vi "Robot Main.vi"() -> ()   [LabVIEW 2019]
doc: "This VI implements the framework and scheduler for your robotics program. It should not be necessary to modify the framework. You are expected to add your code to the VIs called from Robot Main - the ones located in the Team Code folder within the project."
uses:
  <vilib>/Rock Robotics/SystemInterfaces/i2clib/i2c_bus.ctl
panel:
  in  "Color":string(combo)="Red"
  in  "Set Color":bool
  out "Matched Color Name":string
  out "Match Confidence":dbl
  out "Measured Color":cluster{"R":dbl, "G":dbl, "B":dbl}
  in  "Blue Cal":cluster{"R":dbl, "G":dbl, "B":dbl}={"R"=0.143, "G"=0.427, "B"=0.429} caption="Blue Calibration"
  in  "Green Cal":cluster{"R":dbl, "G":dbl, "B":dbl}={"R"=0.197, "G"=0.561, "B"=0.24} caption="Green Calibration"
  in  "Red Cal":cluster{"R":dbl, "G":dbl, "B":dbl}={"R"=0.561, "G"=0.323, "B"=0.114} caption="Red Calibration"
  in  "Yellow Cal":cluster{"R":dbl, "G":dbl, "B":dbl}={"R"=0.361, "G"=0.524, "B"=0.113} caption="Yellow Calibration"
  out "error out":errorcluster
  out "Proximity":u16(graph)
  out "Color":u32(colorbox)
  in  "I2C Bus":T1
  in  "Finish":bool
  # "To save calibration:\n\nEdit --> Make Current Values Default"
  # "------>"
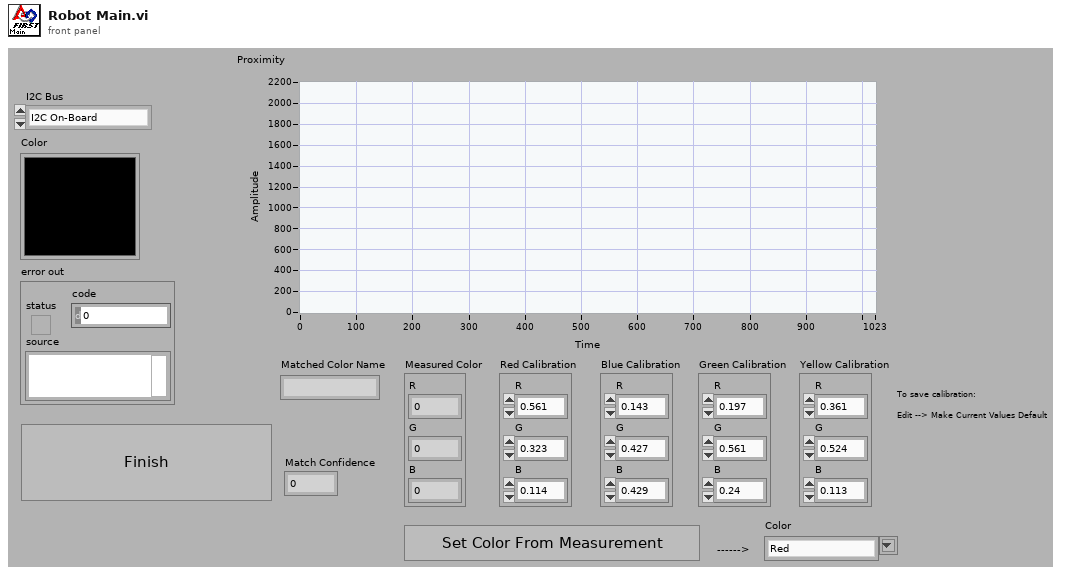
[diagram p1: front panel]
types:
  T1 = typedef "i2c_bus.ctl" = enum16{"I2C On-Board", "I2C MXP", "Invalid"}
  T2 = typedef "Color Sensor V3 DevRef.ctl" = cluster{"I2CDevRef":T3}
  T3 = typedef "WPI_I2CDevRef.ctl" = cluster{"DevStatus":errorcluster, "Device Address":u8, "Handle":i32, "I2C Bus":T1}
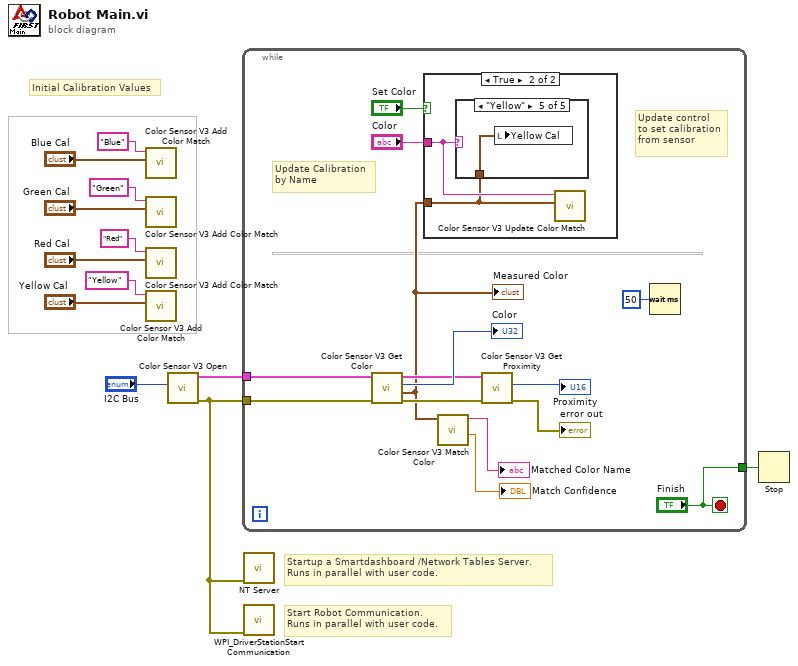
[diagram p0: block diagram]
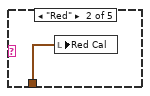
[diagram p4: hidden frame]
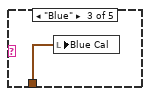
[diagram p5: hidden frame]
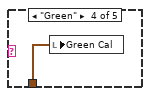
[diagram p6: hidden frame]
diagram:
  # "Initial Calibration Values"
  # "Startup a Smartdashboard /Network Tables Server.\nRuns in parallel with user code."
  # "Start Robot Communication.\nRuns in parallel with user code."
  n1 = call "Color Sensor V3 Add Color Match.vi"("Color"="Blue Cal", "Name"="Blue") -> ()  [unwired: 10 in]
  n2 = call "Color Sensor V3 Add Color Match.vi"("Color"="Green Cal", "Name"="Green") -> ()  [unwired: 10 in]
  n3 = call "Color Sensor V3 Add Color Match.vi"("Color"="Red Cal", "Name"="Red") -> ()  [unwired: 10 in]
  n4 = call "Color Sensor V3 Add Color Match.vi"("Color"="Yellow Cal", "Name"="Yellow") -> ()  [unwired: 10 in]
  n5 = call "Color Sensor V3 Open.vi"("I2C Bus"="I2C Bus") -> ("error out"=w10:errorcluster, "ColorSensorDevRef"=w11:T2)  [unwired: 9 in]
  n6 = while "Scheduling loop" {
    tunnel: w11 -> [w14]
    tunnel: w10 -> [w19]
    tunnel: ["Finish"] -> w9
    stop <- "Finish" stop-if-true
    # "Update control\nto set calibration\nfrom sensor"
    # "Update Calibration\nby Name"
    n7 = call "Color Sensor V3 Get Color.vi"("error in (no error)"=w19, "ColorSensorDevRef"=w14) -> ("error out"=w24:errorcluster, "Normalized Color"=w13:cluster{"R":dbl, "G":dbl, "B":dbl}, "Color"=→"Color":u32, "ColorSensorDevRef out"=w23:T2)  [unwired: 6 in]
    "Measured Color" <- w13
    n8 = case shown="True" "Set Color" {
      tunnel: "Color" -> [_ w28]
      tunnel: w13 -> [_ w27]
      frame False {
      }
      frame True {
        n9 = case shown="\"Yellow\"" w28 {
          tunnel: w27 -> [_ w29 w30 w31 w32]
          frame Default {
          }
          frame "Red" {
            n10 = local write "Red Cal"(w29) -> ()
          }
          frame "Blue" {
            n11 = local write "Blue Cal"(w30) -> ()
          }
          frame "Green" {
            n12 = local write "Green Cal"(w31) -> ()
          }
          frame "Yellow" {
            n13 = local write "Yellow Cal"(w32) -> ()
          }
        }
        n14 = call "Color Sensor V3 Update Color Match.vi"("Color"=w27, "Name"=w28) -> ()  [unwired: 10 in]
      }
    }
    n15 = call "Color Sensor V3 Match Color.vi"("Measured Color"=w13) -> ("Confidence"=→"Match Confidence":dbl, "Matched Color Name"=→"Matched Color Name":string)  [unwired: 8 in, 1 out]
    n16 = call "Color Sensor V3 Get Proximity.vi"("error in (no error)"=w24, "ColorSensorDevRef"=w23) -> ("error out"=→"error out":errorcluster, "Proximity"=→"Proximity":u16)  [unwired: 7 in, 1 out]
    n17 = Wait (ms)(milliseconds to wait=u32 50) -> ()  [unwired: 1 out]
  }
  n18 = call <vilib>:"NT Server.vi"("error in (no error)"=w10) -> ()  [unwired: 11 in]
  n19 = call <vilib>:"WPI_DriverStationStart Communication.vi"("error in (no error)"=w10) -> ()  [unwired: 1 in, 10 out]
  n20 = Stop(stop? (T)=w9) -> ()
